vi "openSession.vi"(8 "error in (no error)":errorcluster caption="entrée d'erreur (pas d'erreur)", 11 "Python en entrée":refnum<class "Python.lvclass">) -> (0 "error out":errorcluster caption="sortie d'erreur", 3 "Python en sortie":refnum<class "Python.lvclass">)   [LabVIEW 2020, in "Python.lvclass"]
doc: "Open a python session"
uses:
  Python.lvclass
  Python.lvclass/Python.ctl
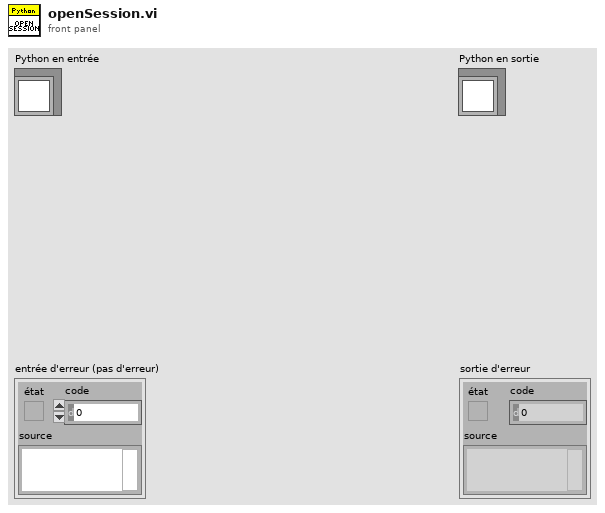
[diagram p1: front panel]
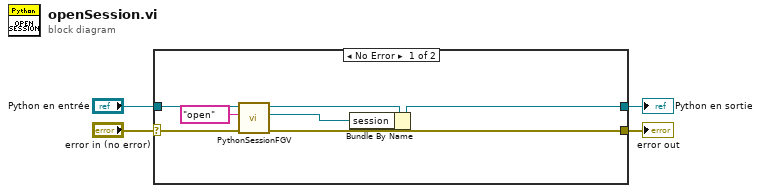
[diagram p0: block diagram]
diagram:
  n1 = case shown="No Error" "error in (no error)" {
    selector: "error in (no error)" -> [w10 w12]
    tunnel: [w5 w12] -> w3
    tunnel: [w6 w11] -> w1
    tunnel: "Python en entrée" -> [w9 w11]
    frame No Error {
      n2 = call "PythonSessionFGV.vi"("error in"=w10, "state"="open") -> ("error out"=w5:errorcluster, "PythonSession"=w7:refnum<k35>)  [unwired: 8 in]
      n3 = Bundle By Name(cluster=w9, "session"=w7) -> (w6:refnum<class "Python.lvclass">)
    }
    frame Error {
    }
  }
  "error out" <- w3
  "Python en sortie" <- w1
